vi "Write.vi"(8 "Error In":errorcluster, 10 "Anything":variant, 11 "Writer In":refnum<class "Writer.lvclass">) -> (0 "Error Out":errorcluster, 3 "Writer Out":refnum<class "Writer.lvclass">)   [LabVIEW 2017, in "LabPack.lvlib"]
uses:
  LabPack.lvlib
  Public/Writer/Writer.lvclass
  Public/Writer/Private/Begin Array by Value.vi
  Public/Writer/Private/End Array by Value.vi
  <vilib>/Utility/Data Type/NI_Data Type.lvlib
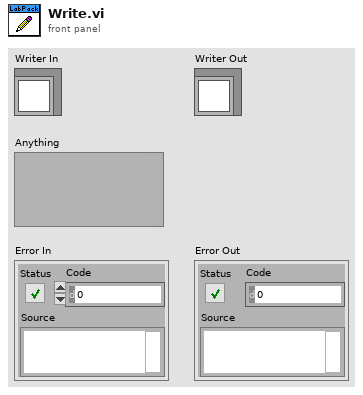
[diagram p1: front panel]
types:
  T1 = typedef "NI_Data Type.lvlib/Data Type.ctl" = enum8{"Invalid Type", "Void", "I8", "I16", "I32", "I64", "U8", "U16", "U32", "U64", "Single Float", "Double Float", "Extended Float", "Single Complex", "Double Complex", "Extended Complex", "Enum U8", "Enum U16", "Enum U32", "Enum U64", "Single Float With Unit", "Double Float With Unit", "Extended Float With Unit", "Single Complex with Unit", "Double Complex with Unit", "Extended Complex with Unit", "Boolean", "String", "Path", "Picture", "Tag", "Array", "Cluster", "Variant", "LV Variant", "Waveform", "Timestamp", "Digital Waveform", "Digital Data", "ExpressData", "Refnum", "External Data", "VI", "Poly VI", "LabVIEW Class Instance", "Fixed Point"}
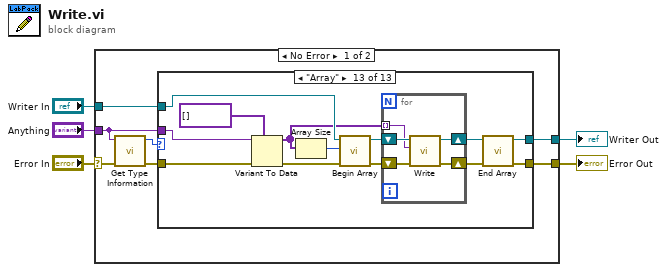
[diagram p0: block diagram]
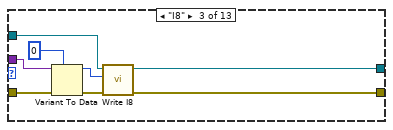
[diagram p4: hidden frame]
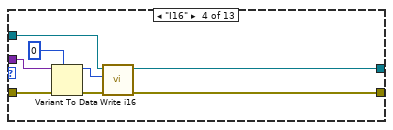
[diagram p5: hidden frame]
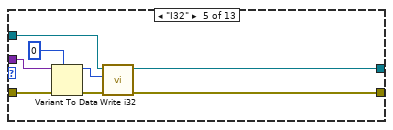
[diagram p6: hidden frame]
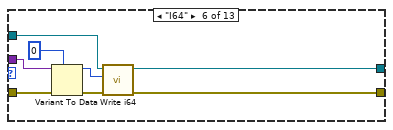
[diagram p7: hidden frame]
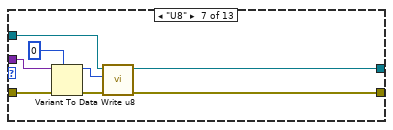
[diagram p8: hidden frame]
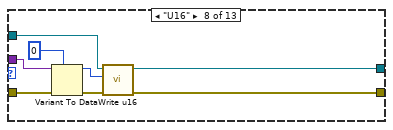
[diagram p9: hidden frame]
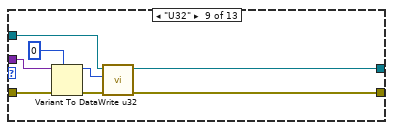
[diagram p10: hidden frame]
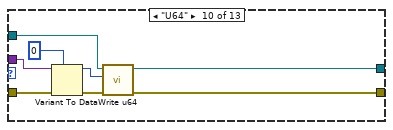
[diagram p11: hidden frame]
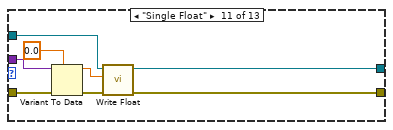
[diagram p12: hidden frame]
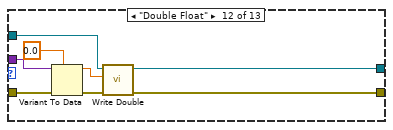
[diagram p13: hidden frame]
diagram:
  n1 = case shown="No Error" "Error In" {
    selector: "Error In" -> [w6 w115]
    tunnel: "Anything" -> [w12 _]
    tunnel: "Writer In" -> [w11 w116]
    tunnel: [w10 w116] -> w3
    tunnel: [w9 w115] -> w2
    frame No Error {
      n2 = call <vilib>:"Get Type Information.vi"("error in (no error)"=w6, "Variant"=w12) -> ("error out"=w8:errorcluster, "Type"=w7:T1)  [unwired: 5 in, 3 out]
      n3 = case shown="\"Array\"" w7 {
        tunnel: w8 -> [w13 w16 w24 w32 w40 w48 w56 w64 w72 w80 w88 w96 w102]
        tunnel: [w13 w16 w18 w26 w34 w42 w50 w58 w66 w74 w82 w90 w107] -> w9
        tunnel: [w14 w15 w20 w28 w36 w44 w52 w60 w68 w76 w84 w92 w108] -> w10
        tunnel: w11 -> [w14 w15 w23 w31 w39 w47 w55 w63 w71 w79 w87 w95 w109]
        tunnel: w12 -> [_ _ w22 w30 w38 w46 w54 w62 w70 w78 w86 w94 w100]
        frame "Invalid Type", Default {
        }
        frame "Void" {
        }
        frame "I8" {
          n4 = Variant To Data(error in=w24, type=i8 0, Variant=w22) -> (data=w17:i8, error out=w19:errorcluster)
          n5 = call "Write I8.vi"("Error In"=w19, "Value"=w17, "Writer In"=w23) -> ("Error Out"=w18:errorcluster, "Writer Out"=w20:refnum<class "Writer.lvclass">)  [unwired: 7 in]
        }
        frame "I16" {
          n6 = Variant To Data(error in=w32, type=i16 0, Variant=w30) -> (data=w25:i16, error out=w27:errorcluster)
          n7 = call "Write i16.vi"("Error In"=w27, "Value"=w25, "Writer In"=w31) -> ("Error Out"=w26:errorcluster, "Writer Out"=w28:refnum<class "Writer.lvclass">)  [unwired: 7 in]
        }
        frame "I32" {
          n8 = Variant To Data(error in=w40, type=0, Variant=w38) -> (data=w33:i32, error out=w35:errorcluster)
          n9 = call "Write i32.vi"("Error In"=w35, "Value"=w33, "Writer In"=w39) -> ("Error Out"=w34:errorcluster, "Writer Out"=w36:refnum<class "Writer.lvclass">)  [unwired: 7 in]
        }
        frame "I64" {
          n10 = Variant To Data(error in=w48, type=i64 0, Variant=w46) -> (data=w41:i64, error out=w43:errorcluster)
          n11 = call "Write i64.vi"("Error In"=w43, "Value"=w41, "Writer In"=w47) -> ("Error Out"=w42:errorcluster, "Writer Out"=w44:refnum<class "Writer.lvclass">)  [unwired: 7 in]
        }
        frame "U8" {
          n12 = Variant To Data(error in=w56, type=u8 0, Variant=w54) -> (data=w49:u8, error out=w51:errorcluster)
          n13 = call "Write u8.vi"("Error In"=w51, "Value"=w49, "Writer In"=w55) -> ("Error Out"=w50:errorcluster, "Writer Out"=w52:refnum<class "Writer.lvclass">)  [unwired: 7 in]
        }
        frame "U16" {
          n14 = Variant To Data(error in=w64, type=u16 0, Variant=w62) -> (data=w57:u16, error out=w59:errorcluster)
          n15 = call "Write u16.vi"("Error In"=w59, "Value"=w57, "Writer In"=w63) -> ("Error Out"=w58:errorcluster, "Writer Out"=w60:refnum<class "Writer.lvclass">)  [unwired: 7 in]
        }
        frame "U32" {
          n16 = Variant To Data(error in=w72, type=u32 0, Variant=w70) -> (data=w65:u32, error out=w67:errorcluster)
          n17 = call "Write u32.vi"("Error In"=w67, "Value"=w65, "Writer In"=w71) -> ("Error Out"=w66:errorcluster, "Writer Out"=w68:refnum<class "Writer.lvclass">)  [unwired: 7 in]
        }
        frame "U64" {
          n18 = Variant To Data(error in=w80, type=u64 0, Variant=w78) -> (data=w73:u64, error out=w75:errorcluster)
          n19 = call "Write u64.vi"("Error In"=w75, "Value"=w73, "Writer In"=w79) -> ("Error Out"=w74:errorcluster, "Writer Out"=w76:refnum<class "Writer.lvclass">)  [unwired: 7 in]
        }
        frame "Single Float" {
          n20 = Variant To Data(error in=w88, type=sgl 0.0, Variant=w86) -> (data=w81:sgl, error out=w83:errorcluster)
          n21 = call "Write Float.vi"("Error In"=w83, "Value"=w81, "Writer In"=w87) -> ("Error Out"=w82:errorcluster, "Writer Out"=w84:refnum<class "Writer.lvclass">)  [unwired: 7 in]
        }
        frame "Double Float" {
          n22 = Variant To Data(error in=w96, type=0.0, Variant=w94) -> (data=w89:dbl, error out=w91:errorcluster)
          n23 = call "Write Double.vi"("Error In"=w91, "Value"=w89, "Writer In"=w95) -> ("Error Out"=w90:errorcluster, "Writer Out"=w92:refnum<class "Writer.lvclass">)  [unwired: 7 in]
        }
        frame "Array" {
          n24 = Variant To Data(error in=w102, type=variant[] [], Variant=w100) -> (data=w98:variant[], error out=w101:errorcluster)
          n25 = Array Size(array=w98) -> (size(s)=w97:i32)
          n26 = call-poly "Begin Array.vi"("Error In"=w101, "Elements Count"=w97, "Writer In"=w109) -> ("Error Out"=w103:errorcluster, "Writer Out"=w106:refnum<class "Writer.lvclass">)  [unwired: 7 in]
          n27 = for {
            shift-right: [w113] -> w105
            shift-left: w106 -> [w114]
            shift-right: [w112] -> w104
            shift-left: w103 -> [w111]
            tunnel: w98 -> [w110] mode=indexing
            n28 = call "Write.vi"("Error In"=w111, "Anything"=w110, "Writer In"=w114) -> ("Error Out"=w112:errorcluster, "Writer Out"=w113:refnum<class "Writer.lvclass">)  [unwired: 7 in]
          }
          n29 = call-poly "End Array.vi"("Error In"=w104, "Writer In"=w105) -> ("Error Out"=w107:errorcluster, "Writer Out"=w108:refnum<class "Writer.lvclass">)  [unwired: 8 in]
        }
      }
    }
    frame Error {
    }
  }
  "Writer Out" <- w3
  "Error Out" <- w2
